vi "Accelerometer Data to Waveform.vi"(11 "Accelerometer Data":T1) -> (2 "accel plot":waveform(dbl)[](array[waveform]), 3 "gyro plot":waveform(dbl)[](array[waveform]))   [LabVIEW 2012]
uses:
  Accelerometer Data.ctl
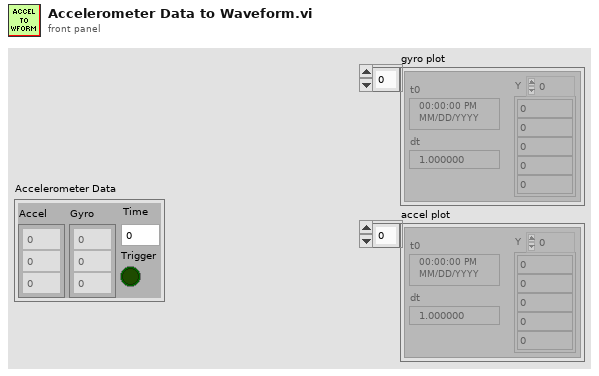
[diagram p1: front panel]
types:
  T1 = typedef "Accelerometer Data.ctl" = cluster{"Accel":dbl[], "Gyro":dbl[], "Time":u64, "Trigger":bool}
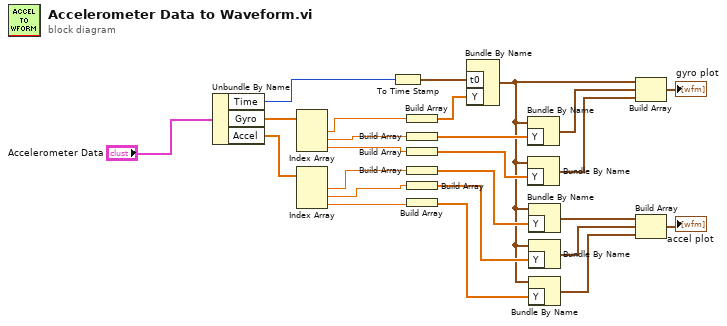
[diagram p0: block diagram]
diagram:
  n1 = Unbundle By Name("Accelerometer Data") -> ("Time"=w24:u64, "Gyro"=w8:dbl[], "Accel"=w4:dbl[])
  n2 = Index Array(array=w8) -> (element #1=w7:dbl, element #2=w6:dbl, element #3=w5:dbl)  [unwired: 3 in]
  n3 = Index Array(array=w4) -> (element #1=w3:dbl, element #2=w2:dbl, element #3=w1:dbl)  [unwired: 3 in]
  n4 = To Time Stamp(1:w24) -> (0:w23:timestamp)
  n5 = Build Array(w7) -> (w22:dbl[])
  n6 = Build Array(w6) -> (w21:dbl[])
  n7 = Build Array(w5) -> (w20:dbl[])
  n8 = Build Array(w3) -> (w19:dbl[])
  n9 = Build Array(w2) -> (w18:dbl[])
  n10 = Build Array(w1) -> (w17:dbl[])
  n11 = Bundle By Name("t0"=w23, "Y"=w22) -> (w9:waveform(dbl))  [unwired: 1 in]
  n12 = Bundle By Name(cluster=w9, "Y"=w21) -> (w16:waveform(dbl))
  n13 = Bundle By Name(cluster=w9, "Y"=w20) -> (w15:waveform(dbl))
  n14 = Bundle By Name(cluster=w9, "Y"=w19) -> (w14:waveform(dbl))
  n15 = Bundle By Name(cluster=w9, "Y"=w18) -> (w13:waveform(dbl))
  n16 = Bundle By Name(cluster=w9, "Y"=w17) -> (w12:waveform(dbl))
  n17 = Build Array(w9, w16, w15) -> (→"gyro plot":waveform(dbl)[])
  n18 = Build Array(w14, w13, w12) -> (→"accel plot":waveform(dbl)[])
